vi "Climber_Globals.vi"() -> ()   [LabVIEW 2020]
uses:
  Subsystems/Climber/Climber_Cluster.ctl
  Subsystems/Climber/Climber_Control_States.ctl
  <vilib>/Rock Robotics/WPI/Solenoid/WPI_SolenoidValue.ctl
panel:
  in  "Air_Brake_Solenoid_Value":T1
  in  "Inner_Arm_Pivot_Motor_Value":dbl
  in  "Outer_Arm_Elevator_Motor_Value":dbl
  in  "Outer_Arm_Pivot_Motor_Value":dbl
  in  "Climber_Execute_Notifier":refnum<notifier>
  in  "Climber_Determiner_Notifier":refnum<notifier>
  in  "Climber_Execute_Ref":string="Climber_Execute_Ref"
  in  "Climber_Determiner_Ref":string="Climber_Determiner_Ref"
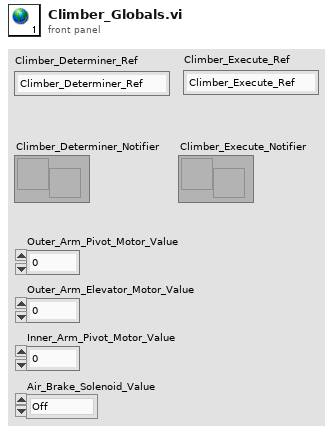
[diagram p1: front panel]
types:
  T1 = typedef "WPI_SolenoidValue.ctl" = enum16{"Off", "On", "Forward", "Reverse"}
diagram:
